vi "test_VISA Read.vi"(8 "error in (no error)":errorcluster, 11 "TestCase in":refnum<class "Serial Protocols Tests.lvclass">) -> (0 "error out":errorcluster, 3 "TestCase out":refnum<class "Serial Protocols Tests.lvclass">)   [LabVIEW 2018, in "Serial Protocols Tests.lvclass"]
uses:
  Serial Protocols Tests.lvclass
  VISA/VISA.lvclass
  C:/Dev/niveristand-instrument-addon-classes/Source/Protocols/Protocol Parent/Protocol Parent.lvclass
  Listener/Listener.lvclass
  Listener/ListenerClassControls/Operation.ctl
  Protocol Parent/Methods/Read Parameter.ctl
  <vilib>/Platform/TimedLoop/XDataNode/timing_clust.ctl
  <vilib>/Platform/TimedLoop/XDataNode/nitl_modes.ctl
  <vilib>/Platform/TimedLoop/XDataNode/wakeup.ctl
  Listener/Listener.lvclass/Listener.ctl
  VISA/VISA.lvclass/VISA.ctl
  <vilib>/platform/TimedLoop/XDataNode/XDataNode.xnode
  <vilib>/addons/_JKI Toolkits/VI Tester/TestCase.llb/TestCase.lvclass
  Protocol Parent/Protocol Parent.lvclass
  <vilib>/Platform/TimedLoop/XDataNode/XDNodeRunTimeDep.lvlib
  C:/Program Files (x86)/National Instruments/LabVIEW 2018/vi.lib/addons/_JKI Toolkits/VI Tester/TestCase.llb/TestCase.lvclass
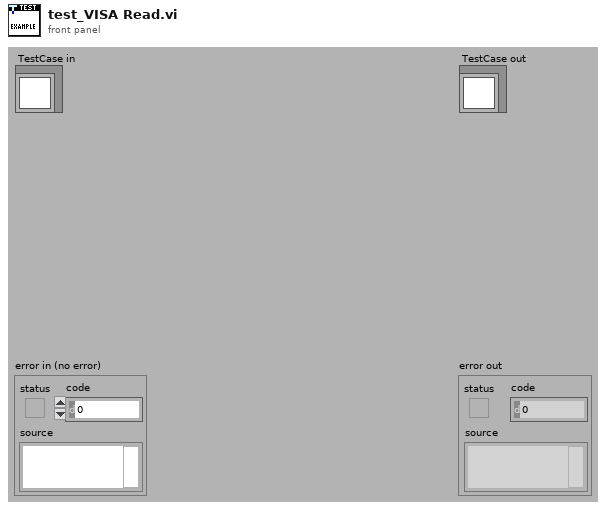
[diagram p1: front panel]
types:
  T1 = typedef "Protocols.lvlib/Protocol Parent.lvclass/Read Parameter.ctl" = cluster{"Wait Type":enum16{"Byte Count", "Wait sec"}, "Wait Value":dbl}
  T2 = typedef "Listener.lvclass/Operation.ctl" = enum16{"Read", "Write"}
  T3 = typedef "XDNodeRunTimeDep.lvlib/timing_clust.ctl" = cluster{"Expected End [f-1]":u64, "Actual End [f-1]":u64, "Finished Late? [f-1]":bool, "Expected End [i-1]":u64, "Actual End [i-1]":u64, "Finished Late? [i-1]":bool, "Expected Start [i]":u64, "Actual Start [i]":u64, "Expected Start [f]":u64, "Actual Start [f]":u64, "Source Name":string, "Structure Name":string, "Period":i64, "Deadline":i64, "Offset":i64, "Start":i64, "Priority":i32, "Timeout":i32, "Mode":T4, "Wakeup Reason":T5, "Error":errorcluster, "Source Type":string, "Secondary Source Type":string, "Global End Time":u64, "Global Start Time":u64, "Frame Duration":u64, "Iteration Duration":u64, "Assigned CPU":i32, "I/O Scan Engine Mode":u32}
  T4 = typedef "XDNodeRunTimeDep.lvlib/nitl_modes.ctl" = enum32{"No Change", "Process missed periods, maintain original phase", "Discard missed periods, maintain original phase", "Process missed periods, ignore original phase", "Discard missed periods, ignore original phase"}
  T5 = typedef "XDNodeRunTimeDep.lvlib/wakeup.ctl" = enum32{"Normal", "Aborted", "Asynchronous wakeup", "Timing source error", "Timed loop error", "Timeout"}
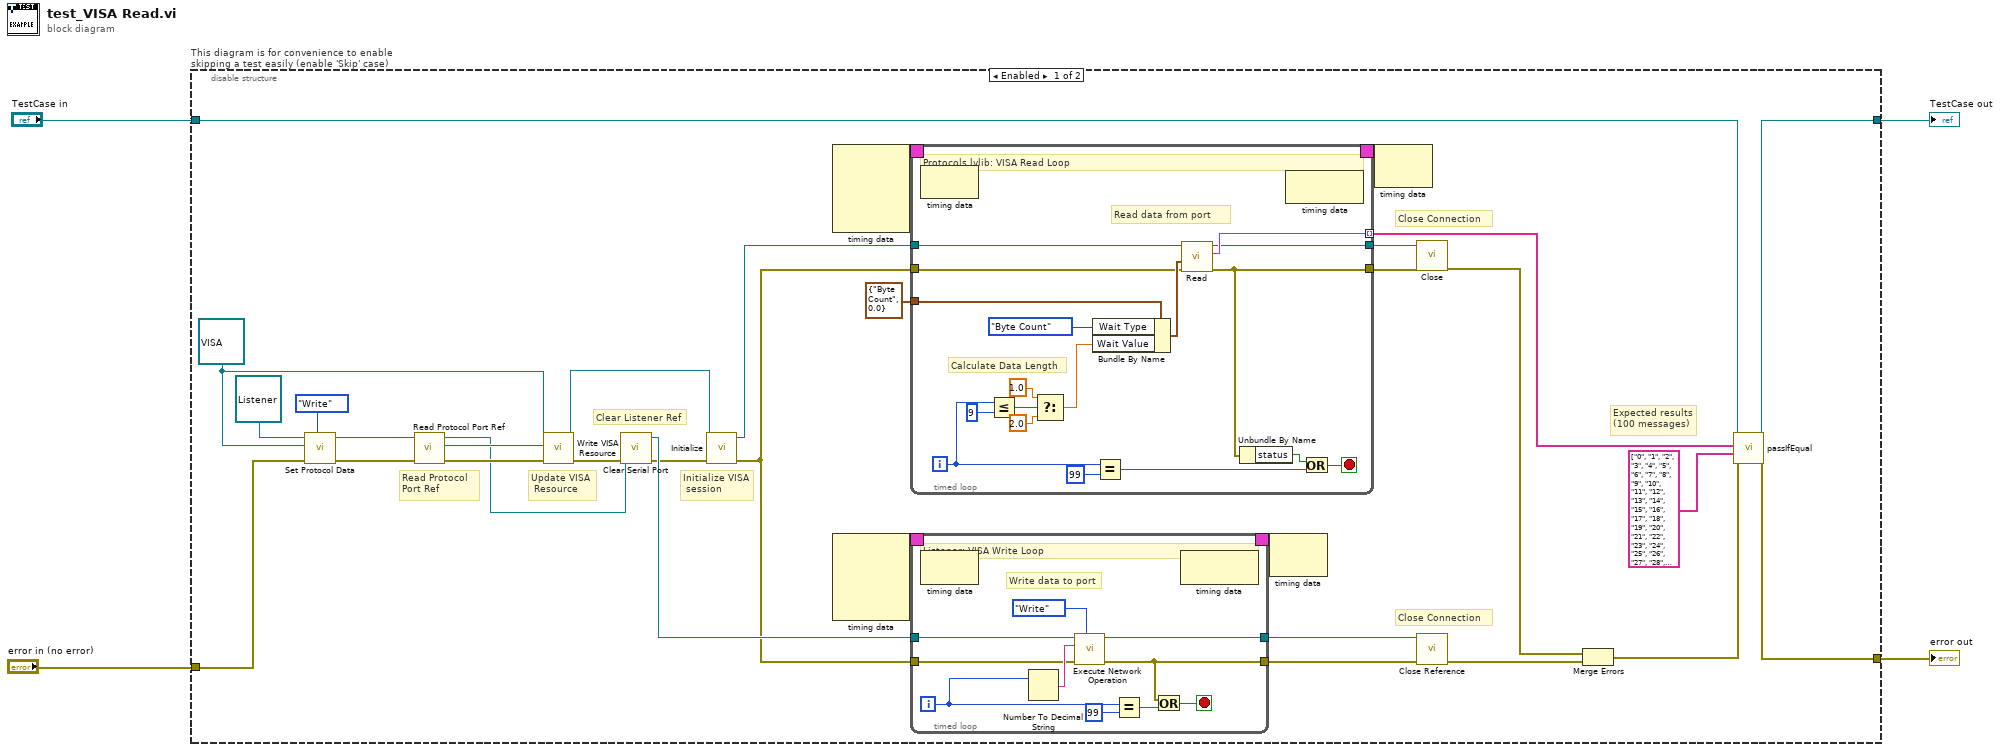
[diagram p0: block diagram]
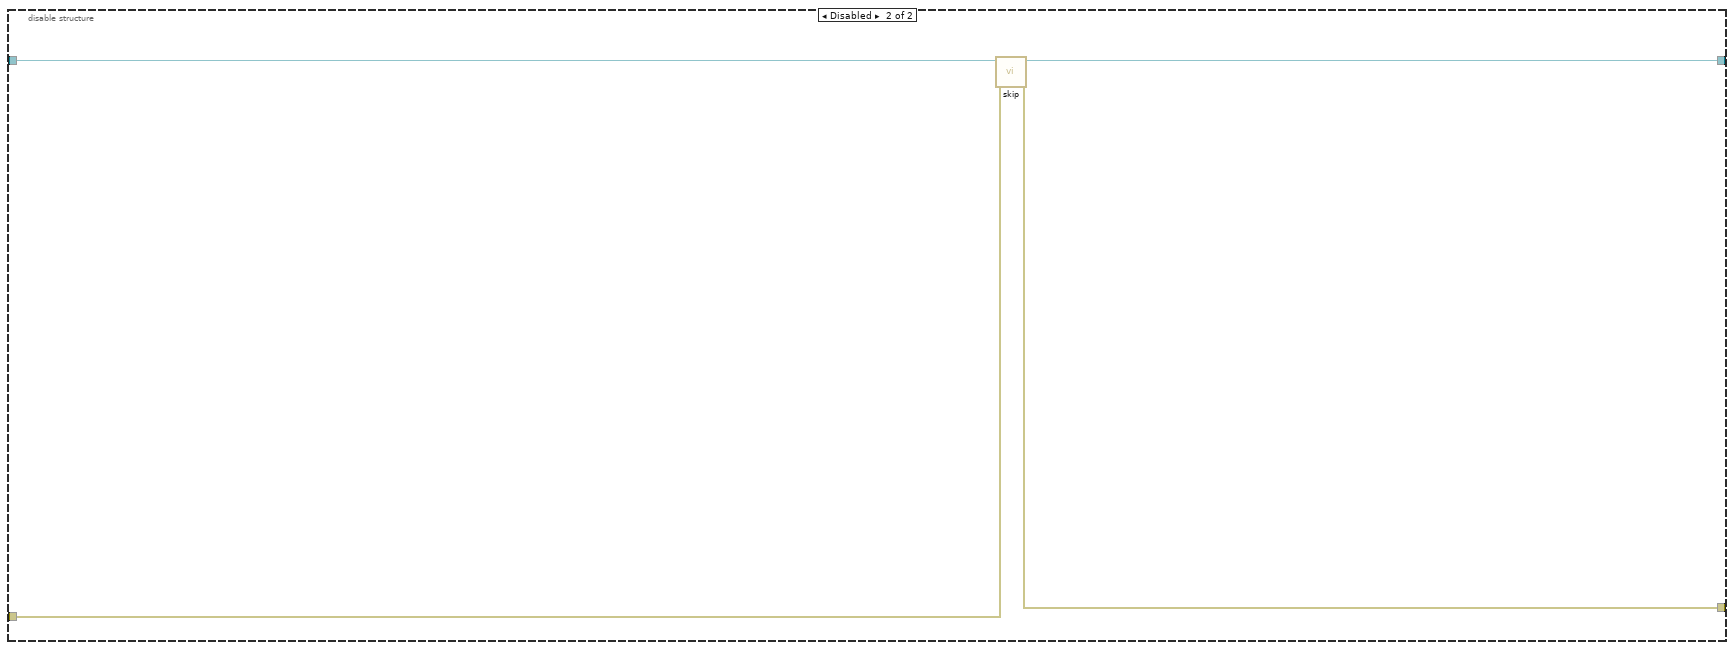
[diagram p2: hidden frame]
diagram:
  n1 = disable-structure "This diagram is for convenience to enable skipping a test easily (enable 'Skip' case)" shown="Enabled" {
    disable-tunnel: "TestCase in" -> [w36 w76]
    disable-tunnel: [w35 w74] -> w1
    disable-tunnel: [w34 w75] -> w3
    disable-tunnel: "error in (no error)" -> [w26 w73]
    frame Enabled {
      w6 = refnum<class "VISA.lvclass"> refnum ("Protocols.lvlib:VISA.lvclass")
      # "Read Protocol \nPort Ref"
      # "Clear Listener Ref"
      # "Close Connection"
      # "Expected results\n(100 messages)"
      # "Close Connection"
      # "Initialize VISA\n session"
      # "Update VISA\n Resource"
      n2 = call "Set Protocol Data.vi"("Operation"=Operation."Write", "error in (no error)"=w26, "Protocols.lvlib:Protocol Parent.lvclass"=w6, "Listener In.lvclass"=refnum<class "Listener.lvclass"> refnum ("Listener.lvclass")) -> ("error out"=w10:errorcluster, "Listener Out.lvclass"=w9:refnum<class "Listener.lvclass">)  [unwired: 6 in]
      n3 = call "Read Protocol Port Ref.vi"("error in (no error)"=w10, "Listener in"=w9) -> ("error out"=w8:errorcluster, "Protocol Port Ref"=w7:refnum<visa-resource-name>, "Listener out"=w5:refnum<class "Listener.lvclass">)  [unwired: 7 in]
      n4 = call "Write VISA Resource.vi"("error in (no error)"=w8, "VISA Resource"=w7, "VISA in"=w6) -> ("error out"=w20:errorcluster, "VISA out"=w19:refnum<class "VISA.lvclass">)  [unwired: 7 in]
      n5 = call "Clear Serial Port.vi"("error in (no error)"=w20, "Listener In.lvclass"=w5) -> ("error out"=w13:errorcluster, "Listener out"=w14:refnum<class "Listener.lvclass">)  [unwired: 8 in]
      n6 = call-dynamic "Initialize.vi"("error in (no error)"=w13, "VISA in"=w19) -> ("error out"=w12:errorcluster, "VISA out"=w21:refnum<class "VISA.lvclass">)  [unwired: 8 in]
      n7 = node-c288() -> (w18:T3)  [unwired: 4 in]
      n8 = node-c288() -> (w16:T3)  [unwired: 4 in]
      n9 = timed-loop {
        tunnel: w12 -> [w59]
        tunnel: [w65] -> w27 mode=indexing
        tunnel: [w55] -> w32
        tunnel: T1 {"Wait Type"=enum."Byte Count", "Wait Value"=0.0} ("Read Parameter") -> [w58]
        timing: w18 -> [_]
        timing-out: [_] -> w17
        tunnel: w21 -> [w60]
        tunnel: [w64] -> w31
        i -> [w56]
        stop <- w61 stop-if-true
        # "Calculate Data Length"
        # "Read data from port"
        # "Protocols.lvlib: VISA Read Loop"
        n10 = node-c288() -> ()  [unwired: 1 in, 1 out]
        n11 = Less Or Equal?(x=w56, y=9) -> (x <= y?=w53:bool)
        n12 = Select(t=1.0 ("Wait Value"), s=w53, f=2.0) -> (s? t:f=w50:dbl)
        n13 = Bundle By Name(cluster=w58, "Wait Type"=enum16{"Byte Count", "Wait sec"}."Byte Count", "Wait Value"=w50) -> (w66:T1)
        n14 = Equal?(x=w56, y=99) -> (x = y?=w62:bool)
        n15 = call-dynamic "Read.vi"("error in (no error)"=w59, "Variant"=w66, "VISA in"=w60) -> ("error out"=w55:errorcluster, "String"=w65:string, "VISA out"=w64:refnum<class "VISA.lvclass">)  [unwired: 6 in]
        n16 = Unbundle By Name(w55) -> ("status"=w54:bool)
        n17 = node-c288() -> ()  [unwired: 1 in, 1 out]
        n18 = Or(x=w54, y=w62) -> (x .or. y?=w61:bool)
      }
      n19 = timed-loop {
        tunnel: [w42] -> w24
        timing: w16 -> [_]
        timing-out: [_] -> w15
        tunnel: w12 -> [w37]
        tunnel: w14 -> [w46]
        tunnel: [w45] -> w23
        i -> [w39]
        stop <- w41 stop-if-true
        # "Write data to port"
        # "Listener: VISA Write Loop"
        n20 = node-c288() -> ()  [unwired: 1 in, 1 out]
        n21 = Number To Decimal String(number=w39) -> (decimal integer string=w40:string)  [unwired: 1 in]
        n22 = call "Execute Network Operation.vi"("Operation"=Operation."Write", "error in (no error)"=w37, "Message"=w40, "Listener In.lvclass"=w46) -> ("error out"=w42:errorcluster, "Listener Out.lvclass"=w45:refnum<class "Listener.lvclass">)  [unwired: 6 in]
        n23 = Equal?(x=w39, y=99) -> (x = y?=w43:bool)
        n24 = Or(x=w42, y=w43) -> (x .or. y?=w41:bool)
        n25 = node-c288() -> ()  [unwired: 1 in, 1 out]
      }
      n26 = node-c288(w15) -> ()  [unwired: 1 out]
      n27 = node-c288(w17) -> ()  [unwired: 1 out]
      n28 = call-dynamic "Close.vi"("error in (no error)"=w32, "VISA in"=w31) -> ("error out"=w29:errorcluster)  [unwired: 8 in, 1 out]
      n29 = call "Close Reference.vi"("error in (no error)"=w24, "Listener In.lvclass"=w23) -> ("error out"=w22:errorcluster)  [unwired: 8 in, 1 out]
      n30 = Merge Errors(w29, w22) -> (w28:errorcluster)
      n31 = call-dynamic "passIfEqual.vi"("error in (no error)"=w28, "y"=string[] ["0", "1", "2", "3", "4", "5", "6", "7", "8", "9", "10", "11", "12", "13", "14", "15", "16", "17", "18", "19", "20", "21", "22", "23", "24", "25", "26", "27", "28", "29", "30", "31", "32", "33", "34", "35", "36", "37", "38", "39", "40", "41", "42", "43", "44", "45", "46", "47", "48", "49", "50", "51", "52", "53", "54", "55", "56", "57", "58", "59", "60", "61", "62", "63", "64", "65", "66", "67", "68", "69", "70", "71", "72", "73", "74", "75", "76", "77", "78", "79", "80", "81", "82", "83", "84", "85", "86", "87", "88", "89", "90", "91", "92", "93", "94", "95", "96", "97", "98", "99"] ("Array"), "x"=w27, "TestCase in"=w36) -> ("error out"=w34:errorcluster, "TestCase out"=w35:refnum<class "Serial Protocols Tests.lvclass">)  [unwired: 6 in]
    }
    frame Disabled {
      # "skip test result while test is under development"
      n32 = call <vilib>:"skip.vi"("error in (no error)"=w73, "TestCase in"=w76) -> ("error out"=w75:errorcluster, "TestCase out"=w74:refnum<class "Serial Protocols Tests.lvclass">)  [unwired: 8 in]
    }
  }
  "error out" <- w3
  "TestCase out" <- w1
